vi "Match Multiple Patterns.vi"(4 "Advanced Options":cluster{"Item":u16, "Value":dbl}[](array[cluster]) {"Item" items=["LD Sampling - Minimum Constrast"=0, "LD Sampling - Enable Subpixel Accuracy"=1, "LD Sampling - Search Strategy"=2, "LD Sampling - Subpixel Iterations"=3, "LD Sampling - Subpixel Tolerance"=4, "LD Sampling - Initial Match List Length"=5, "LD Sampling - Match List Reduction Factor"=6, "LD Sampling - Initial Step Size"=7, "LD Sampling - Intermediate Angular Accuracy"=8, "-"=9, "Pyramid - Max Pyramid Level"=100, "Pyramid - Minimum Contrast"=102, "Pyramid - Enable Subpixel Accuracy"=103, "Pyramid - Subpixel Iterations"=104, "Pyramid - Subpixel Tolerance"=105, "Pyramid - Initial Match List Length"=106, "Pyramid - Match List Reduction Factor"=107, "Pyramid - Intermediate Angular Accuracy"=108, "Pyramid - Process Border Matches"=109, "Pyramid - Min Match Separation Distance"=111, "Pyramid - Min Match Separation Angle"=112, "Pyramid - Max Match Overlap"=113, "Pyramid - Max Cache in MB"=114, "Pyramid - Clear Cache"=115]}, 6 "Parameters":T3={"Number of Matches Requested"=1, "Minimum Match Score"=800.0, "Angle Ranges"=[]}, 7 "Algorithm":i32(ring)=2 items=["All", "Low Discrepancy Sampling", "Grayscale Value Pyramid", "Gradients Pyramid"], 8 "error in (no error)":errorcluster, 9 "ROI Descriptor":T2 {"Contours"."Type" items=["No Selection", "Point", "Line", "Rectangle", "Oval", "Polygon", "Freehand Region", "Annulus", "Unused2", "Unused3", "Broken Line", "Freehand Line", "Rotated Rectangle"]}, 10 "Image":T4, 11 "MultiPattern Matcher in":refnum<class "MultiPattern Matcher.lvclass">) -> (0 "error out":errorcluster, 2 "Filtered Matches":T1(array[cluster]), 3 "MultiPattern Matcher out":refnum<class "MultiPattern Matcher.lvclass">)   [LabVIEW 2013, in "MultiPattern Matcher.lvclass"]
uses:
  MultiPattern Matcher.lvclass
  <vilib>/vision/Image Controls.llb/IMAQ Image.ctl
  MultiPattern Matcher.lvclass/MultiPattern Matcher.ctl
  <vilib>/vision/NI_Vision_Development_Module.lvlib
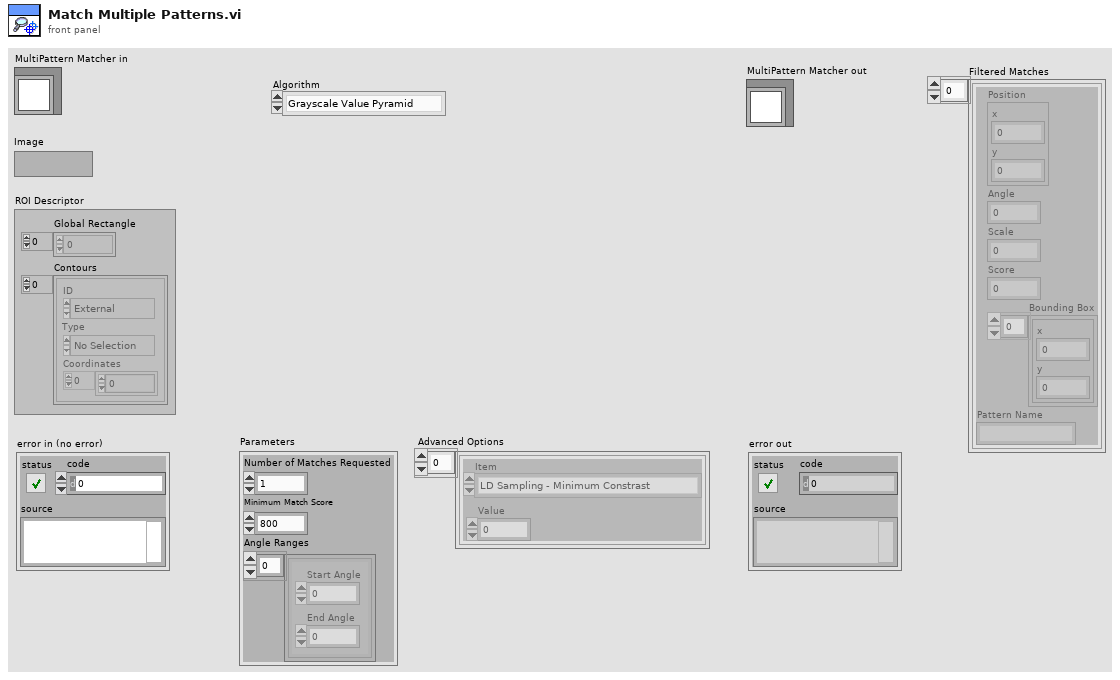
[diagram p1: front panel]
types:
  T1 = cluster{"Position":cluster{"x":sgl, "y":sgl}, "Angle":sgl, "Scale":sgl, "Score":sgl, "Bounding Box":cluster{"x":sgl, "y":sgl}[], "Pattern Name":string}[]
  T2 = typedef "ROI Descriptor" = cluster{"Global Rectangle":i32[], "Contours":cluster{"ID":enum32{"External", "Internal"}, "Type":u32, "Coordinates":i32[]}[]}
  T3 = cluster{"Number of Matches Requested":i32, "Minimum Match Score":sgl, "Angle Ranges":cluster{"Start Angle":sgl, "End Angle":sgl}[]}
  T4 = typedef "IMAQ Image.ctl" = refnum<image>
  T5 = cluster{"Position":cluster{"x":sgl, "y":sgl}, "Angle":sgl, "Scale":sgl, "Score":sgl, "Bounding Box":cluster{"x":sgl, "y":sgl}[], "Pattern Name":string}
  T6 = cluster{"Position":cluster{"x":sgl, "y":sgl}, "Angle":sgl, "Scale":sgl, "Score":sgl, "Bounding Box":cluster{"x":sgl, "y":sgl}[]}[]
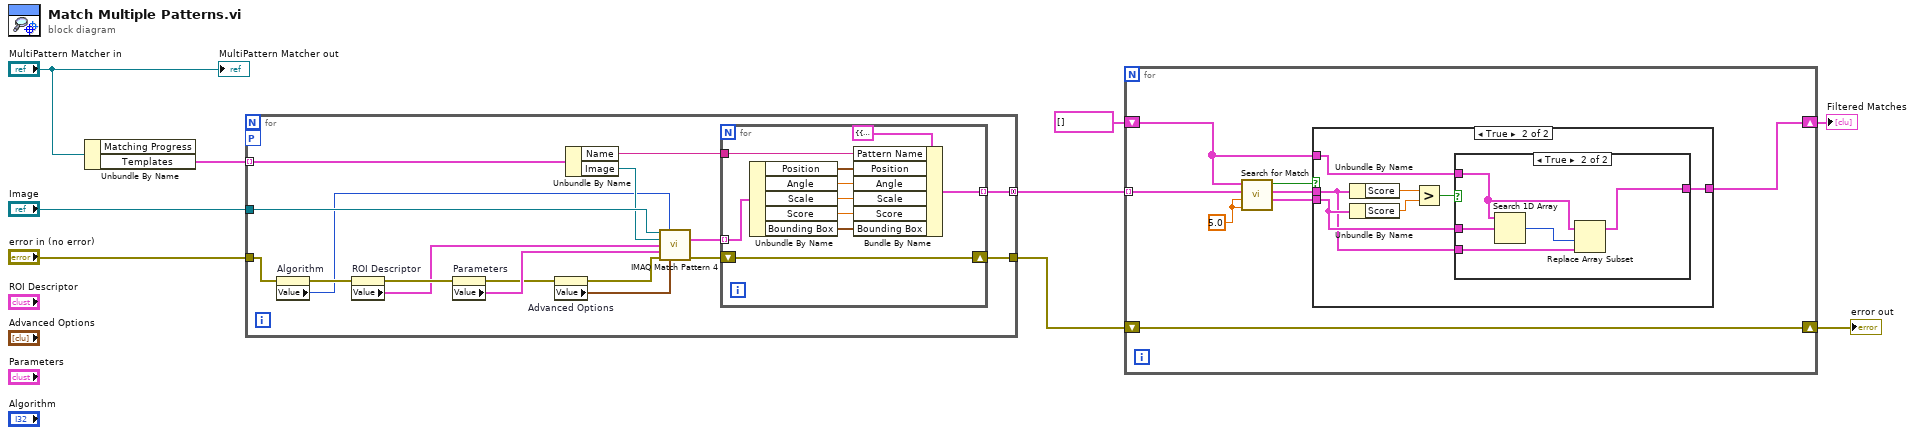
[diagram p0: block diagram]
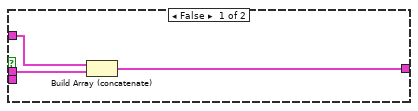
[diagram p2: hidden frame]
diagram:
  n1 = Unbundle By Name("MultiPattern Matcher in") -> ("Templates"=w6:cluster{"Image":T4, "Name":string}[])  [unwired: 1 out]
  n2 = for {
    tunnel: "Image" -> [w25]
    tunnel: w6 -> [w26] mode=indexing
    workers-P: _ -> [_]
    tunnel: "error in (no error)" -> [w10]
    tunnel: [w12] -> w4
    tunnel: [w11] -> w5 mode=concatenating
    n3 = property on="Algorithm" class="Ring (strict)"(error in=w10) -> (error out=w17:errorcluster, "Value"=w16:i32)  [unwired: 1 in, 1 out]
    n4 = property on="ROI Descriptor" class="Clust (strict)"(error in=w17) -> (error out=w23:errorcluster, "Value"=w18:T2)  [unwired: 1 in, 1 out]
    n5 = property on="Parameters" class="Clust (strict)"(error in=w23) -> (error out=w21:errorcluster, "Value"=w22:T3)  [unwired: 1 in, 1 out]
    n6 = property on="Advanced Options" class="Arr (strict)"(error in=w21) -> (error out=w20:errorcluster, "Value"=w19:cluster{"Item":u16, "Value":dbl}[])  [unwired: 1 in, 1 out]
    n7 = Unbundle By Name(w26) -> ("Name"=w14:string, "Image"=w24:T4)
    n8 = call "IMAQ Match Pattern 4"("Image"=w25, "Algorithm"=w16, "Template Image"=w24, "ROI Descriptor"=w18, "Parameters"=w22, "error in (no error)"=w20, "Advanced Options"=w19) -> ("Matches (pixel)"=w15:T6, "error out"=w13:errorcluster)  [unwired: 4 in, 3 out]
    n9 = for {
      tunnel: w15 -> [w36] mode=indexing
      tunnel: w14 -> [w34]
      tunnel: [w28] -> w11 mode=indexing
      shift-right: [w27] -> w12
      shift-left: w13 -> [w27]
      n10 = Unbundle By Name(w36) -> ("Position"=w33:cluster{"x":sgl, "y":sgl}, "Angle"=w32:sgl, "Scale"=w31:sgl, "Score"=w30:sgl, "Bounding Box"=w29:cluster{"x":sgl, "y":sgl}[])
      n11 = Bundle By Name(cluster=T5 {"Position"={"x"=0.0, "y"=0.0}, "Angle"=0.0, "Scale"=0.0, "Score"=0.0, "Bounding Box"=[], "Pattern Name"=""} ("element"), "Pattern Name"=w34, "Position"=w33, "Angle"=w32, "Scale"=w31, "Score"=w30, "Bounding Box"=w29) -> (w28:T5)
    }
  }
  n12 = for {
    tunnel: w5 -> [w38] mode=indexing
    shift-right: [w41] -> w1
    shift-left: T1 [] -> [w42]
    shift-right: [w40] -> w2
    shift-left: w4 -> [w40]
    w37 = sgl 5.0 ("dx")
    n13 = call "Search for Match.vi"("dy"=w37, "dx"=w37, "Match"=w38, "Matches"=w42) -> ("Existing Match"=w39:T5, "Match (duplicate)"=w43:T5, "Match in Matches?"=w44:bool)  [unwired: 5 in]
    n14 = case shown="True" w44 {
      tunnel: w43 -> [w47 w48]
      tunnel: w42 -> [w46 w51]
      tunnel: [w45 w50] -> w41
      tunnel: w39 -> [_ w49]
      frame False {
        n15 = Build Array (concatenate)(w46, w47) -> (w45:T1)
      }
      frame True {
        n16 = Unbundle By Name(w48) -> ("Score"=w54:sgl)
        n17 = Unbundle By Name(w49) -> ("Score"=w53:sgl)
        n18 = Greater?(x=w54, y=w53) -> (0:w52:bool)
        n19 = case shown="True" w52 {
          tunnel: w51 -> [w55 w57]
          tunnel: [w55 w56] -> w50
          tunnel: w49 -> [_ w59]
          tunnel: w48 -> [_ w58]
          frame False {
          }
          frame True {
            n20 = Search 1D Array(1D array=w57, element=w59) -> (index of element=w60:i32)  [unwired: 1 in]
            n21 = Replace Array Subset(array=w57, new element=w58, index=w60) -> (w56:T1)
          }
        }
      }
    }
  }
  "error out" <- w2
  "Filtered Matches" <- w1
  "MultiPattern Matcher out" <- "MultiPattern Matcher in"
